vi "Google Earth - Streaming info.vi"(8 "error in":errorcluster, 11 "Refnum in":refnum<k7>) -> (0 "error out":errorcluster, 1 "StreamingProgressPercentage":i32, 2 "ElevationExaggeration":dbl, 3 "Refnum Out":refnum<k7>, 5 "AutoPilotSpeed":dbl)   [LabVIEW 2009]
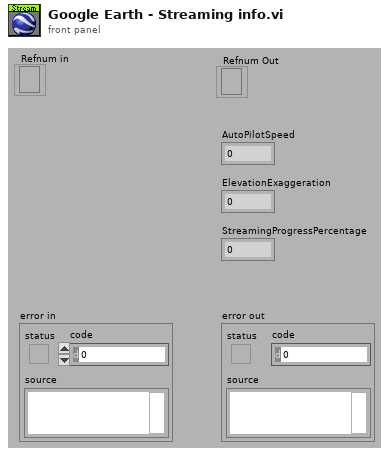
[diagram p1: front panel]
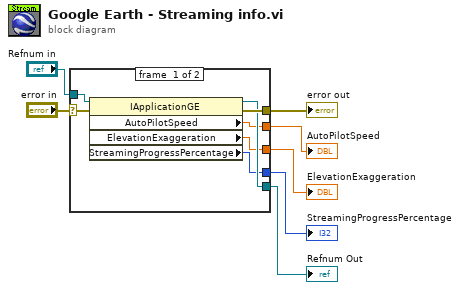
[diagram p0: block diagram]
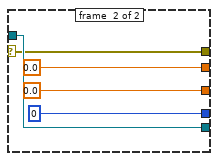
[diagram p2: hidden frame]
diagram:
  n1 = case shown="Error" "error in" {
    selector: "error in" -> [w8 w18]
    tunnel: [w14 w18] -> w7
    tunnel: [w13 w19] -> w6
    tunnel: "Refnum in" -> [w12 w19]
    tunnel: [w11 0 ("StreamingProgressPercentage")] -> w4
    tunnel: [w10 0.0 ("ElevationExaggeration")] -> w3
    tunnel: [w9 0.0 ("AutoPilotSpeed")] -> w2
    frame #0 {
      n2 = property class="IApplicationGE"(reference=w12, error in=w8) -> (reference out=w13:refnum<k7>, error out=w14:errorcluster, "AutoPilotSpeed"=w9:dbl, "ElevationExaggeration"=w10:dbl, "StreamingProgressPercentage"=w11:i32)
    }
    frame #1 {
    }
  }
  "error out" <- w7
  "Refnum Out" <- w6
  "StreamingProgressPercentage" <- w4
  "ElevationExaggeration" <- w3
  "AutoPilotSpeed" <- w2
